vi "IPI_mmToPluse.vi"(10 "X Radio":string, 11 "mm":dbl) -> (0 "Pluse":dbl, 3 "Pluse":string)   [LabVIEW 2015]
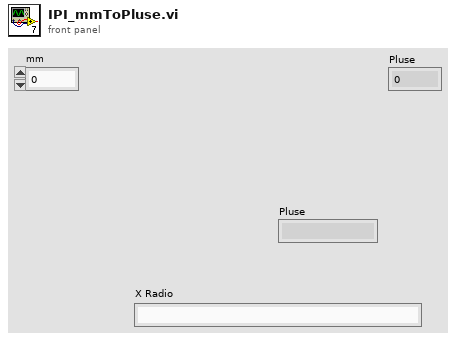
[diagram p1: front panel]
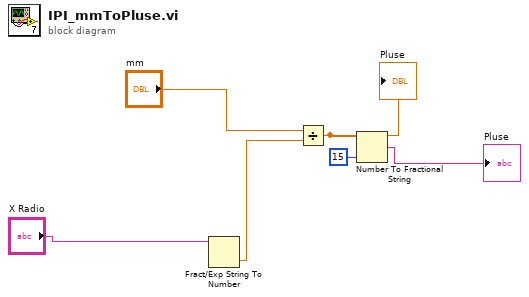
[diagram p0: block diagram]
diagram:
  n1 = Fract/Exp String To Number(string="X Radio") -> (number=w6:dbl)  [unwired: 3 in, 1 out]
  n2 = Divide(x="mm", y=w6) -> (x/y=w5:dbl)
  "Pluse" <- w5
  n3 = Number To Fractional String(number=w5, precision (6)=i16 15 ("精度(6)")) -> (F-format string=→"Pluse":string)  [unwired: 2 in]
